vi "LIA Frequency Shift Simulator.vi"() -> ()   [LabVIEW 2017]
uses:
  <instrlib>/_niInstr/DSP/v1/Shared/Public/IQ Data.ctl
  <vilib>/measure/maspectr.llb/FFT Power Spectrum and PSD for 1 Chan (CDB).vi
  <instrlib>/_niInstr/DSP/v1/FPGA/Public/Sub VIs/Frequency Shift/Frequency Shift - 1 spc.vi
  <instrlib>/_niInstr/DSP/v1/Xnodes/Public/Frequency Shift/niInstr DSP v1 Frequency Shift FPGA.xnode
  <vilib>/Analysis/NI_AALBase.lvlib
  <vilib>/measure/NI_MAPro.lvlib
  <instrlib>/_niInstr/DSP/v1/Shared/niInstr DSP v1 Shared.lvlib
  <instrlib>/_niInstr/DSP/v1/FPGA/niInstr DSP v1 FPGA.lvlib
panel:
  out "logical AND":bool
  out "size(s)":i32
  out "Numeric":i32
  out "Waveform Graph 3":dbl[][](graph)
  out "Waveform Graph 2":cluster{"f0":dbl, "df":dbl, "magnitude":dbl[]}(graph)
  out "Waveform Graph":cluster{"f0":dbl, "df":dbl, "magnitude":dbl[]}(graph)
  in  "Sampling Rate":dbl=1.0 format="%#_p"
  out "FFT Gain":dbl
  out "Noise (W|50ohms)":dbl
  out "k":dbl
  out "Noise vrms":dbl
  in  "Desired SNR (dB)":dbl format="%#_p"
  in  "Oscillator Magnitude":dbl=1.0 format="%#_13g"
  in  "Oscillator Frequency":dbl=0.001 format="%#_p"
  in  "Signal Offset":cdb format="%#_13g"
  in  "Singal Amplitude":dbl=0.5 format="%#_13g"
  in  "Signal Frequency":dbl=0.001 format="%#_p"
  in  "Number Samples":i32=16384
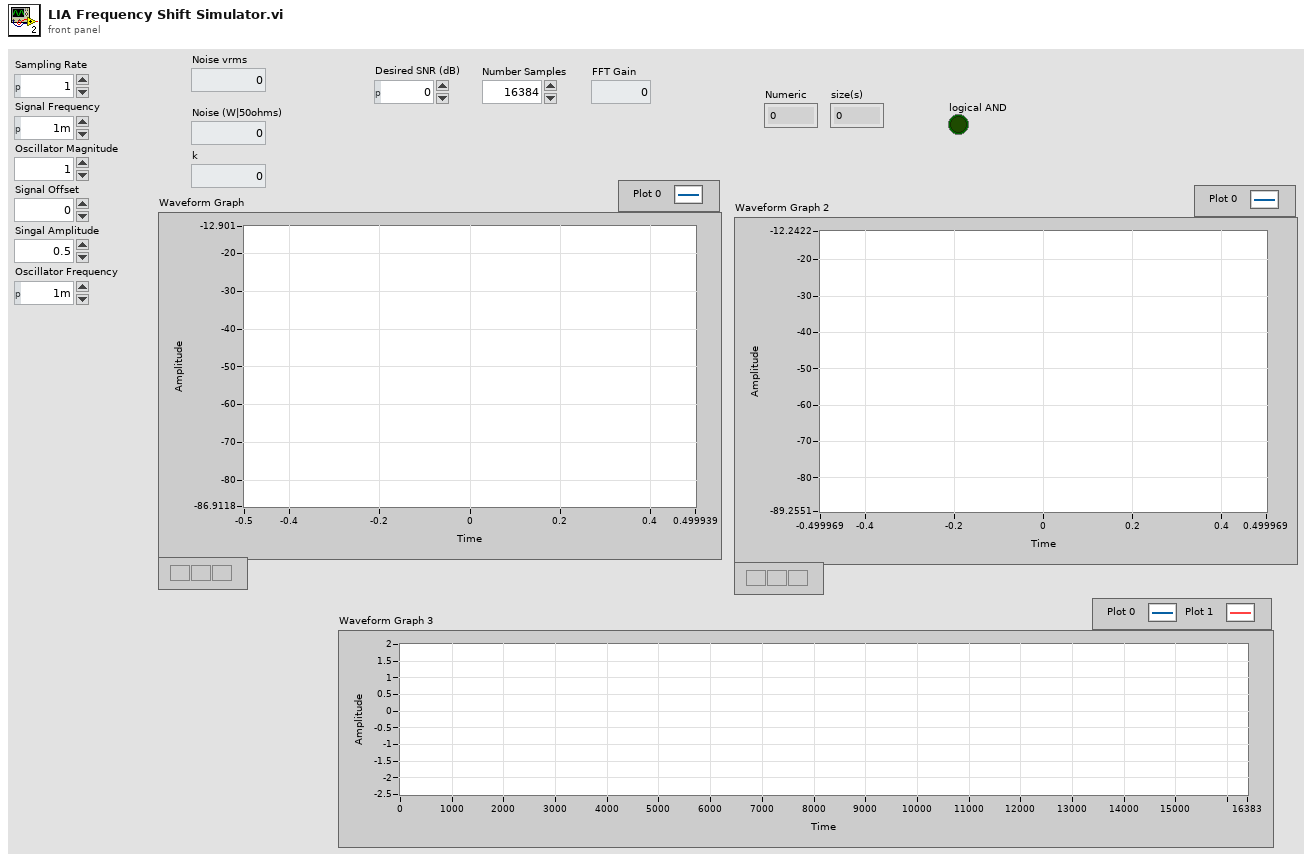
[diagram p1: front panel]
types:
  T1 = typedef "niInstr DSP v1 Shared.lvlib/IQ Data.ctl" = cluster{"I":fxp<+/-,18,1>, "Q":fxp<+/-,18,1>, "overflow":bool}
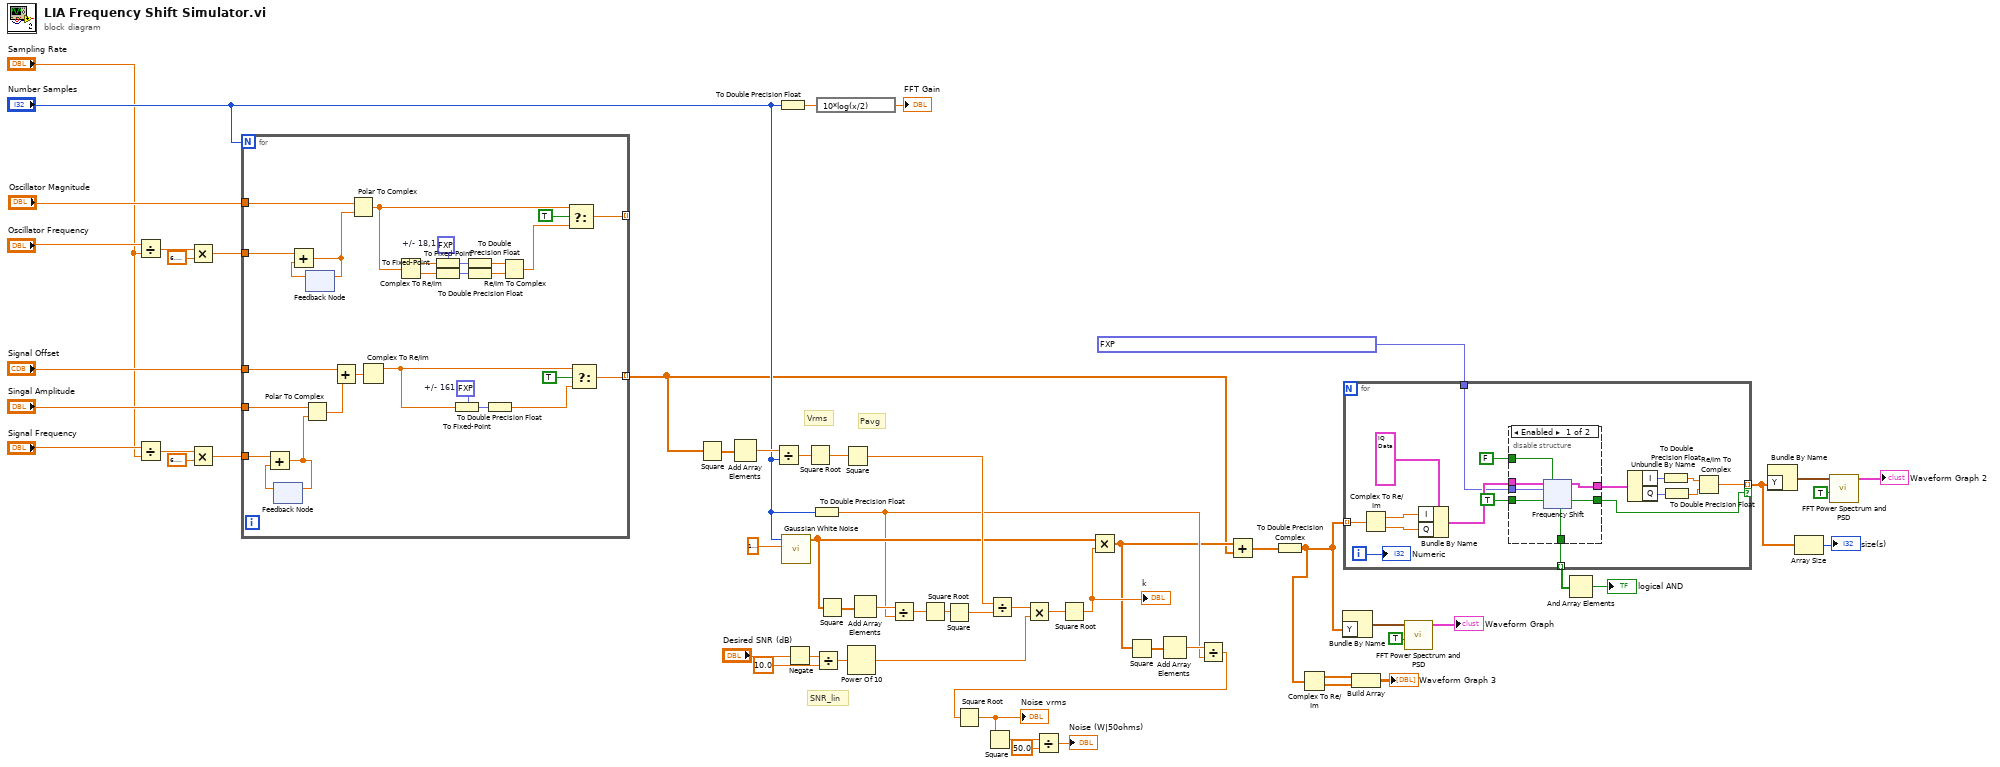
[diagram p0: block diagram]
diagram:
  # "SNR_lin"
  # "Pavg"
  # "Vrms"
  n1 = Divide(x="Oscillator Frequency", y="Sampling Rate") -> (x/y=w55:dbl)
  n2 = Divide(x="Signal Frequency", y="Sampling Rate") -> (x/y=w59:dbl)
  n3 = Multiply(x=w55, y=6.283185307179586) -> (x*y=w52:dbl)
  n4 = Multiply(x=w59, y=6.283185307179586) -> (x*y=w58:dbl)
  n5 = for {
    N: "Number Samples" -> [_]
    tunnel: w58 -> [w85]
    tunnel: "Singal Amplitude" -> [w88]
    tunnel: "Signal Offset" -> [w87]
    tunnel: [w71] -> _ mode=indexing
    tunnel: [w65] -> w17 mode=indexing
    tunnel: w52 -> [w76]
    tunnel: "Oscillator Magnitude" -> [w74]
    w66 = fxp<+/-,16,1> 0.0  # +/- 161
    w81 = fxp<+/-,18,1> 0.0  # +/- 18,1
    n6 = feedback #1() -> (w89:dbl)  [unwired: 1 in]
    n7 = Add(x=w85, y=w89) -> (x+y=w84:dbl)
    n8 = feedback-in #1(w84) -> ()
    n9 = Polar To Complex(1:w84, 2:w88) -> (0:w86:cdb)
    n10 = feedback #2() -> (w75:dbl)  [unwired: 1 in]
    n11 = Add(x=w76, y=w75) -> (x+y=w73:dbl)
    n12 = feedback-in #2(w73) -> ()
    n13 = Add(x=w87, y=w86) -> (x+y=w63:cdb)
    n14 = Polar To Complex(1:w73, 2:w74) -> (0:w72:cdb)
    n15 = Complex To Re/Im(x + iy=w63) -> (x=w62:dbl)  [unwired: 1 out]
    n16 = Complex To Re/Im(x + iy=w72) -> (x=w83:dbl, y=w82:dbl)
    n17 = To Fixed-Point(fixed-point type=w81, number=w83) -> (fixed-point=w80:fxp<+/-,18,1>)
    n18 = To Fixed-Point(fixed-point type=w81, number=w82) -> (fixed-point=w79:fxp<+/-,18,1>)
    n19 = To Fixed-Point(fixed-point type=w66, number=w62) -> (fixed-point=w67:fxp<+/-,16,1>)
    n20 = To Double Precision Float(number=w80) -> (double precision float=w78:dbl)
    n21 = To Double Precision Float(number=w79) -> (double precision float=w77:dbl)
    n22 = To Double Precision Float(number=w67) -> (double precision float=w64:dbl)
    n23 = Re/Im To Complex(1:w77, 2:w78) -> (0:w70:cdb)
    n24 = Select(t=w72, s=TRUE, f=w70) -> (s? t:f=w71:cdb)
    n25 = Select(t=w62, s=TRUE, f=w64) -> (s? t:f=w65:dbl)
  }
  n26 = Square(x=w17) -> (x^2=w50:dbl[])
  n27 = Add Array Elements(numeric array=w50) -> (sum=w49:dbl)
  n28 = Divide(x=w49, y="Number Samples") -> (x/y=w48:dbl)
  n29 = To Double Precision Float(number="Number Samples") -> (double precision float=w22:dbl)
  n30 = call <vilib>:"Gaussian White Noise.vi"("standard deviation"=1.0000000000000002, "samples"="Number Samples") -> ("Gaussian noise pattern"=w32:dbl[])  [unwired: 8 in, 1 out]
  n31 = Negate(x="Desired SNR (dB)") -> (-x=w35:dbl)
  n32 = Square Root(x=w48) -> (sqrt(x)=w47:dbl)
  n33 = To Double Precision Float(number="Number Samples") -> (double precision float=w20:dbl)
  n34 = Divide(x=w35, y=10.0) -> (x/y=w43:dbl)
  n35 = expression code="10*log(x/2)"(w22) -> (→"FFT Gain":dbl)
  n36 = Square(x=w32) -> (x^2=w39:dbl[])
  n37 = Square(x=w47) -> (x^2=w38:dbl)
  n38 = Power Of 10(x=w43) -> (10^x=w34:dbl)
  n39 = Add Array Elements(numeric array=w39) -> (sum=w40:dbl)
  n40 = Divide(x=w40, y=w20) -> (x/y=w41:dbl)
  n41 = Square Root(x=w41) -> (sqrt(x)=w42:dbl)
  n42 = Square(x=w42) -> (x^2=w37:dbl)
  n43 = Divide(x=w38, y=w37) -> (x/y=w36:dbl)
  n44 = Multiply(x=w36, y=w34) -> (x*y=w33:dbl)
  n45 = Square Root(x=w33) -> (sqrt(x)=w31:dbl)
  "k" <- w31
  n46 = Multiply(x=w32, y=w31) -> (x*y=w18:dbl[])
  n47 = Square(x=w18) -> (x^2=w30:dbl[])
  n48 = Add Array Elements(numeric array=w30) -> (sum=w29:dbl)
  n49 = Divide(x=w29, y=w20) -> (x/y=w28:dbl)
  n50 = Square Root(x=w28) -> (sqrt(x)=w27:dbl)
  "Noise vrms" <- w27
  n51 = Square(x=w27) -> (x^2=w26:dbl)
  n52 = Divide(x=w26, y=50.0) -> (x/y=→"Noise (W|50ohms)":dbl)
  n53 = Add(x=w18, y=w17) -> (x+y=w16:dbl[])
  n54 = To Double Precision Complex(1:w16) -> (0:w9:cdb[])
  n55 = Complex To Re/Im(x + iy=w9) -> (x=w8:dbl[], y=w7:dbl[])
  n56 = Bundle By Name("Y"=w9) -> (w15:waveform(cdb))  [unwired: 1 in]
  n57 = for {
    tunnel: w9 -> [w105] mode=indexing
    tunnel: [w98] -> w5 mode=indexing if=w91
    tunnel: fxp<+/-,48,0> 0.0010000000000012221 ("frequency shift") -> [w94]
    tunnel: [w90] -> w2 mode=indexing
    i -> [w97]
    n58 = Complex To Re/Im(x + iy=w105) -> (x=w104:dbl, y=w103:dbl)
    n59 = Bundle By Name(cluster=T1 {"I"=0.0, "Q"=0.0, "overflow"=FALSE} ("IQ_Data_In"), "I"=w104, "Q"=w103) -> (w96:T1)
    n60 = disable-structure shown="Enabled" {
      disable-tunnel: w96 -> [w113 _]
      disable-tunnel: FALSE ("reset") -> [w112 _]
      disable-tunnel: w94 -> [w111 _]
      disable-tunnel: [w110 _] -> w93
      disable-tunnel: TRUE ("input valid") -> [w109 _]
      disable-tunnel: [w108 _] -> w91
      disable-tunnel: [w107 _] -> w90
      frame Enabled {
        n61 = xnode "Frequency Shift"("data in"=w113, "reset"=w112, "frequency shift"=w111, "input valid"=w109) -> ("data out"=w110:T1, "output valid"=w108:bool, "ready for input"=w107:bool)  [unwired: 2 in]
      }
      frame Disabled {
      }
    }
    n62 = Unbundle By Name(w93) -> ("I"=w102:fxp<+/-,18,1>, "Q"=w101:fxp<+/-,18,1>)
    n63 = To Double Precision Float(number=w102) -> (double precision float=w100:dbl)
    n64 = To Double Precision Float(number=w101) -> (double precision float=w99:dbl)
    n65 = Re/Im To Complex(1:w99, 2:w100) -> (0:w98:cdb)
    "Numeric" <- w97
  }
  n66 = Build Array(w8, w7) -> (→"Waveform Graph 3":dbl[][])
  n67 = call-poly <vilib>:"FFT Power Spectrum and PSD.vi"("dB On (F)"=TRUE, "time signal"=w15) -> ("Power Spectrum / PSD"=→"Waveform Graph":cluster{"f0":dbl, "df":dbl, "magnitude":dbl[]})  [unwired: 6 in, 3 out]
  n68 = And Array Elements(Boolean array=w2) -> (logical AND=→"logical AND":bool)
  n69 = Bundle By Name("Y"=w5) -> (w10:waveform(cdb))  [unwired: 1 in]
  n70 = Array Size(array=w5) -> (size(s)=→"size(s)":i32)
  n71 = call-poly <vilib>:"FFT Power Spectrum and PSD.vi"("dB On (F)"=TRUE, "time signal"=w10) -> ("Power Spectrum / PSD"=→"Waveform Graph 2":cluster{"f0":dbl, "df":dbl, "magnitude":dbl[]})  [unwired: 6 in, 3 out]
